vi "S2C_FORNAX_Proc_ProcessReturn.vi"(7 "Text":bool, 8 "Error In":errorcluster, 9 "JSON":string, 10 "Return":string, 11 "Command":string) -> (0 "Error Out":errorcluster, 3 "Data":string)   [LabVIEW 2015]
uses:
  PolyDriver/Typedefs/ParameterRangeState.ctl
  PolyDriver/Typedefs/BoardId.ctl
  PolyDriver/Typedefs/BoardIdDataSet.ctl
  PolyDriver/Typedefs/CalibrationType.ctl
  PolyDriver/Typedefs/ExternalCommPairingStatus.ctl
  PolyDriver/Typedefs/DftMode.ctl
  PolyDriver/Typedefs/SystemSettings.ctl
  PolyDriver/Typedefs/UserSettings.ctl
  PolyDriver/Typedefs/SystemState.ctl
  PolyDriver/Typedefs/EnergyChannelId.ctl
  PolyDriver/Typedefs/EnergyModes.ctl
  PolyDriver/Typedefs/SwitchId.ctl
  PolyDriver/Typedefs/SwitchState.ctl
  PolyDriver/Typedefs/SwitchSource.ctl
  S2C_FORNAX_Proc_Globals.vi
panel:
  in  "SwitchSource":T1 items=["SWITCH_SOURCE_UNKNOWN", "SWITCH_SOURCE_HANDSWITCH", "SWITCH_SOURCE_FOOTSWITCH", "SWITCH_SOURCE_AUTO_BIPOLAR", "SWITCH_SOURCE_CARDIOBLATE", "SWITCH_SOURCE_SCREEN", "NUM_SWITCH_SOURCES"]
  in  "SwitchState":T2 items=["SWITCH_STATE_NULL", "SWITCH_STATE_PRESSED", "SWITCH_STATE_RELEASED", "NUM_SWITCH_STATES"]
  in  "SwitchId":T3 items=["SWITCH_ID_NONE", "SWITCH_ID_CUT", "SWITCH_ID_VMODE", "SWITCH_ID_COAG", "SWITCH_ID_LIGASURE", "SWITCH_ID_BIPOLAR", "SWITCH_ID_STAPLER_CLOSE", "SWITCH_ID_STAPLER_OPEN", "SWITCH_ID_CARDIOBLATE_BIPOLAR", "SWITCH_ID_CARDIOBLATE_BIPOLAR_TOUCHSCREEN", "SWITCH_ID_CARDIOBLATE_MONOPOLAR", "SWITCH_ID_CARDIOBLATE_MONOPOLAR_TOUCHSCREEN", "SWITCH_ID_ULTRASONIC_BTN1", "SWITCH_ID_ULTRASONIC_BTN2", "SWITCH_ID_MAX"]
  in  "EnergyModes":T4 items=["SPRAY_MODE"=0, "CUT_MODE"=1, "BLEND_MODE"=2, "FULGERATE_MODE"=3, "BIPOLAR_MODE"=4, "VESSEL_SEALING_MODE"=5, "VALLEYLAB_MODE"=6, "BIPOLAR_RESECTION_CUT_MODE"=7, "BIPOLAR_RESECTION_COAG_MODE"=8, "AUTOBIPOLAR_MODE"=9, "VIPER_HLA"=10, "SOFT_COAG_MODE"=11, "ECUT_MODE"=12, "SHARED_SPRAY_MODE"=13, "SHARED_FULGERATE_MODE"=14, "CARDIO_MONO_MODE"=15, "CARDIO_BIPOLAR_MODE"=16, "BIPOLAR_LOW_MODE"=17, "BIPOLAR_MACRO_MODE"=18, "BIPOLAR_STANDARD_MODE"=19, "BIPOLAR_MEDIUM_MODE"=20, "VL_ENDOSCOPY_MODE"=21, "NUM_ENERGY_MODES"=22, "MODE_NOT_USED"=-1]
  in  "EnergyChannelId":T5 items=["EC_MONO_1"=0, "EC_BIPOLAR"=1, "EC_MONO_2"=2, "EC_ADVANCED"=3, "EC_ADVANCED_ECUT"=4, "EC_ADVANCED_DCUT"=5, "EC_SHARED_COAG"=6, "EC_INTERNAL_BIP_CAL"=7, "EC_NOT_USED"=-1]
  in  "SystemState":T6 items=["SYSTEM_STATE_INVALID", "SYSTEM_STATE_INIT", "SYSTEM_STATE_POST", "SYSTEM_STATE_CLINICAL", "SYSTEM_STATE_SERVICE", "SYSTEM_STATE_SW_UPDATE", "SYSTEM_STATE_SHUTDOWN", "SYSTEM_STATE_CALIBRATION", "SYSTEM_STATE_CONFIGURATION", "SYSTEM_STATE_CLINICAL_CONFIGURATION"]
  in  "UserSettings":T7 items=["USER_SETTINGS_INVALID", "USER_SETTINGS_LANGUAGE", "USER_SETTINGS_VOLUME", "USER_SETTINGS_ALIAS", "USER_SETTINGS_NETWORK_CONFIG", "USER_SETTINGS_AUTO_NETWORK_ON", "USER_SETTINGS_KEYBOARD_LANGUAGE", "NUM_USER_SETTINGS"]
  in  "SystemSettings":T8 items=["SYSTEM_SETTINGS_INVALID", "SYSTEM_SETTINGS_COUNTRY", "SYSTEM_SETTINGS_REGION", "SYSTEM_SETTINGS_BIPOLAR_RESECTION", "SYSTEM_SETTINGS_INSTRUMENT_ID_MODE", "SYSTEM_SETTINGS_SMOKE_EVAC_MODE", "NUM_SYSTEM_SETTINGS"]
  in  "DftMode":T9 items=["DFT_MODE_NONE", "DFT_MODE_PAIRED", "DFT_MODE_DFA", "DFT_MODE_DFT"]
  in  "ExternalCommPairingStatus":T10 items=["EXTERNAL_COMM_PAIRING_STATUS_NOT_AVAILABLE", "EXTERNAL_COMM_PAIRING_STATUS_AVAILABLE", "EXTERNAL_COMM_PAIRING_STATUS_PAIRED", "NUM_EXTERNAL_COMM_PAIRING_STATUS"]
  in  "CalibrationType":T11 items=["CALIBRATION_TYPE_FIELD"=0, "CALIBRATION_TYPE_FACTORY"=1, "CALIBRATION_TYPE_UNKNOWN"=-1]
  in  "BoardIdDataSet":T12 items=["BOARD_ID_DATASET_BOARD_INFO"=0, "BOARD_ID_DATASET_SCHEMA_INFO"=1, "BOARD_ID_DATASET_CHASSIS_INSTALLATION"=2, "BOARD_ID_DATASET_CONFIGURATION"=3, "BOARD_ID_DATASET_CALIBRATION_CURR"=4, "BOARD_ID_DATASET_RESERVED_1"=5, "BOARD_ID_DATASET_RESERVED_2"=6, "BOARD_ID_DATASET_RESERVED_3"=7, "BOARD_ID_DATASET_CALIBRATION_HIST_TOC"=8, "BOARD_ID_DATASET_CALIBRATION_HIST"=9, "BOARD_ID_DATASET_INIT_MAX"=10, "BOARD_ID_DATASET_MAX"=50]
  in  "BoardId":T13 items=["BOARD_ID_NONE", "BOARD_ID_CONTROLLER", "BOARD_ID_STEERING_RELAY", "BOARD_ID_RF", "BOARD_ID_POWER_SUPPLY", "BOARD_ID_FRONT_PANEL", "BOARD_ID_MAX"]
  in  "ParameterRangeState":T14 items=["PARAMETER_RANGE_STATE_UNKNOWN", "PARAMETER_RANGE_STATE_AT_MIN", "PARAMETER_RANGE_STATE_AT_MAX", "PARAMETER_RANGE_STATE_BETWEEN_MINMAX", "PARAMETER_RANGE_STATE_LESS_THAN_MIN", "PARAMETER_RANGE_STATE_GREATER_THAN_MAX"]
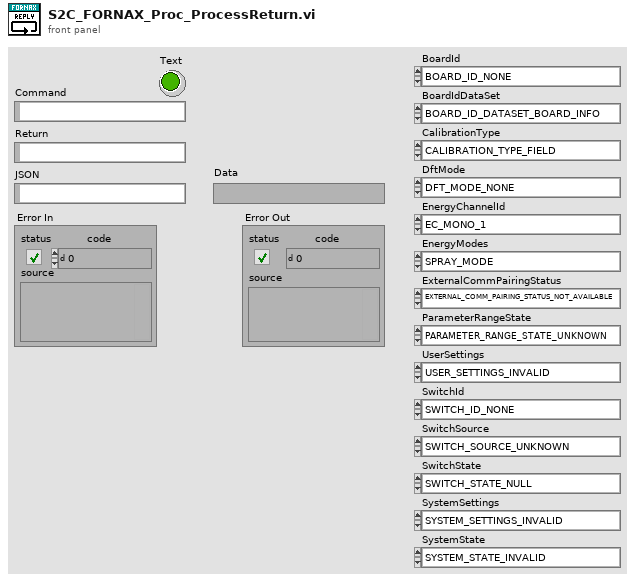
[diagram p1: front panel]
types:
  T1 = typedef "SwitchSource.ctl" = i16
  T2 = typedef "SwitchState.ctl" = i16
  T3 = typedef "SwitchId.ctl" = i16
  T4 = typedef "EnergyModes.ctl" = i16
  T5 = typedef "EnergyChannelId.ctl" = i16
  T6 = typedef "SystemState.ctl" = i16
  T7 = typedef "UserSettings.ctl" = i16
  T8 = typedef "SystemSettings.ctl" = i16
  T9 = typedef "DftMode.ctl" = i16
  T10 = typedef "ExternalCommPairingStatus.ctl" = i16
  T11 = typedef "CalibrationType.ctl" = i16
  T12 = typedef "BoardIdDataSet.ctl" = i16
  T13 = typedef "BoardId.ctl" = i16
  T14 = typedef "ParameterRangeState.ctl" = i16
  T15 = cluster{"Partition":string, "Message":string, "M_BarcodeImageFile":string}
  T16 = cluster{"Partition":string, "Message":string, "M_BoardId":T13, "M_BoardIdDataSet":T12, "M_Value":string, "M_Crc32":i32}
  T17 = cluster{"Partition":string, "Message":string, "M_BoardId":T13, "M_BoardIdDataSet":T12, "M_Value":string}
  T18 = cluster{"Partition":string, "Message":string, "M_EnergyChannelId":T5, "M_CutMode":T4, "M_CutPower":i32, "M_CutPowerRangeState":T14, "M_CoagMode":T4, "M_CoagPower":i32, "M_CoagPowerRangeState":T14, "M_Crc32":i32}
  T19 = cluster{"Partition":string, "Message":string, "M_EnergyChannelId":T5, "M_CutMode":T4, "M_CutPower":i32, "M_CutPowerRangeState":T14, "M_CoagMode":T4, "M_CoagPower":i32, "M_CoagPowerRangeState":T14}
  T20 = cluster{"Partition":string, "Message":string, "M_EnergyChannelId":T5, "M_SourceId":T1, "M_SwitchId":T3, "M_SwitchState":T2, "M_Crc32":i32}
  T21 = cluster{"Partition":string, "Message":string, "M_EnergyChannelId":T5, "M_SourceId":T1, "M_SwitchId":T3, "M_SwitchState":T2}
  T22 = cluster{"Partition":string, "Message":string, "M_CalibrationType":T11, "M_CalibrationTime":string, "M_Options":string, "M_EmA2dCalData.M_MonoLowVoltPrimary.M_Offset":dbl, "M_EmA2dCalData.M_MonoLowVoltPrimary.M_Gain":dbl, "M_EmA2dCalData.M_MonoLowVoltSecondary.M_Offset":dbl, "M_EmA2dCalData.M_MonoLowVoltSecondary.M_Gain":dbl, "M_EmA2dCalData.M_MonoHighVoltPrimary.M_Offset":dbl, "M_EmA2dCalData.M_MonoHighVoltPrimary.M_Gain":dbl, "M_EmA2dCalData.M_MonoHighVoltSecondary.M_Offset":dbl, "M_EmA2dCalData.M_MonoHighVoltSecondary.M_Gain":dbl, "M_EmA2dCalData.M_BipLowVoltPrimary.M_Offset":dbl, "M_EmA2dCalData.M_BipLowVoltPrimary.M_Gain":dbl, "M_EmA2dCalData.M_BipLowVoltSecondary.M_Offset":dbl, "M_EmA2dCalData.M_BipLowVoltSecondary.M_Gain":dbl, "M_EmA2dCalData.M_BipHighVoltPrimary.M_Offset":dbl, "M_EmA2dCalData.M_BipHighVoltPrimary.M_Gain":dbl, "M_EmA2dCalData.M_BipHighVoltSecondary.M_Offset":dbl, "M_EmA2dCalData.M_BipHighVoltSecondary.M_Gain":dbl, "M_EmA2dCalData.M_BipLowCurrentPrimary.M_Offset":dbl, "M_EmA2dCalData.M_BipLowCurrentPrimary.M_Gain":dbl, "M_EmA2dCalData.M_BipLowCurrentSecondary.M_Offset":dbl, "M_EmA2dCalData.M_BipLowCurrentSecondary.M_Gain":dbl, "M_EmA2dCalData.M_BipHighCurrentPrimary.M_Offset":dbl, "M_EmA2dCalData.M_BipHighCurrentPrimary.M_Gain":dbl, "M_EmA2dCalData.M_BipHighCurrentSecondary.M_Offset":dbl, "M_EmA2dCalData.M_BipHighCurrentSecondary.M_Gain":dbl}
  T23 = cluster{"Partition":string, "Message":string, "M_ControllerBoardId":string, "M_ChassisSerialNumber":string, "M_Alias":string, "M_PrimaryIpAddress":string, "M_PairingStatus":T10, "M_PairedEntityIpAddress":string, "M_PairedEntityAlias":string, "M_PairedEntityId":string, "M_Options":string, "M_DftMode":T9, "M_IsViperEnabled":bool}
  T24 = cluster{"Partition":string, "Message":string, "M_DisplayOrder":i32, "M_FeatureSetting":i32, "M_FeatureSettingName":string, "M_FeatureStatus":i32, "M_FeatureStatusText":string, "M_IntValue":i32, "M_IsEnablable":bool, "M_IsEnabled":bool, "M_IsEntitled":bool, "M_IsEntitlable":bool, "M_LastEnabledUpdate":i32, "M_LastEntitledUpdate":i32, "M_LicenseKey":string, "M_LicenseTerms":string, "M_Options":string, "M_StringValue":string}
  T25 = cluster{"Partition":string, "Message":string, "M_SystemSetting":T8, "M_IntValue":i32, "M_StringValue":string}
  T26 = cluster{"Partition":string, "Message":string, "M_UtcTime":string, "M_LocalTime":string, "M_TimeZone":string}
  T27 = cluster{"Partition":string, "Message":string, "M_UserSetting":T7, "M_IntValue":i32, "M_StringValue":string}
  T28 = cluster{"Partition":string, "Message":string, "M_VolumeBars":i32, "M_RangeState":T14, "M_VolumeCloseOverlay":bool}
  T29 = cluster{"Partition":string, "Message":string, "M_ViperMessage":string, "M_SrcId":i32}
  T30 = cluster{"Partition":string, "Message":string, "M_message":string, "M_srcId":i32}
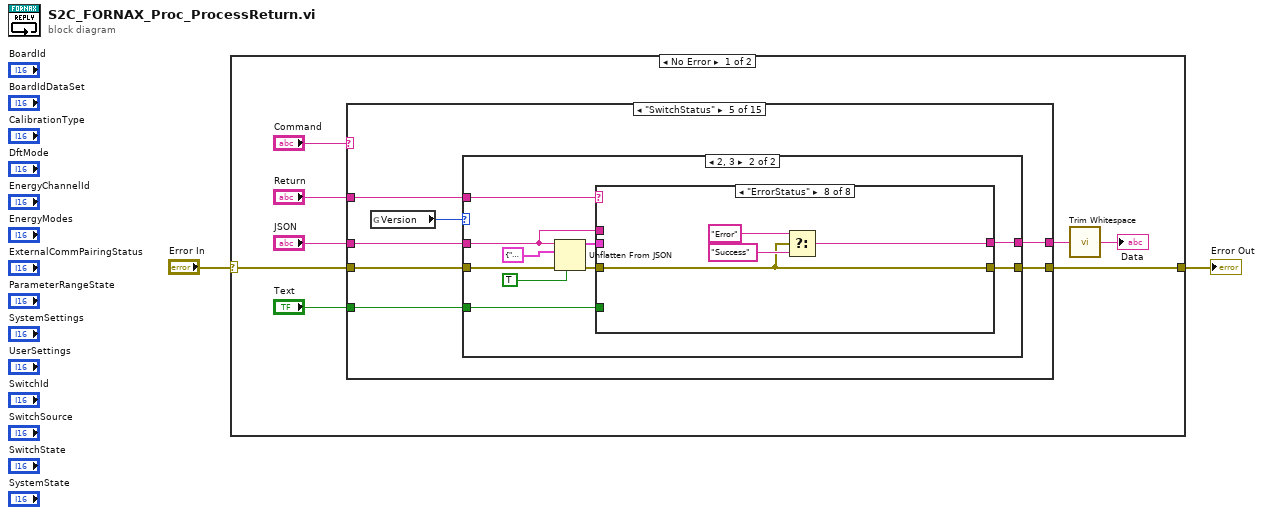
[diagram p0: block diagram]
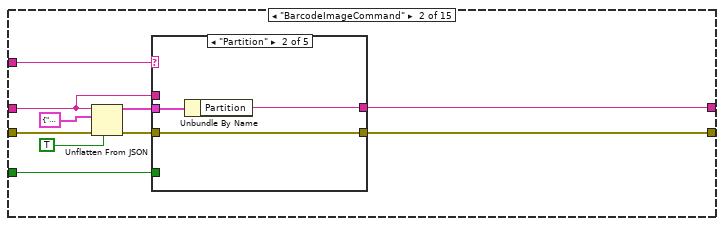
[diagram p3: hidden frame]
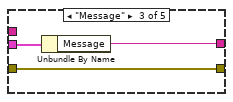
[diagram p5: hidden frame]
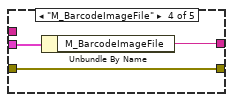
[diagram p6: hidden frame]
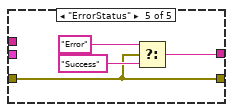
[diagram p7: hidden frame]
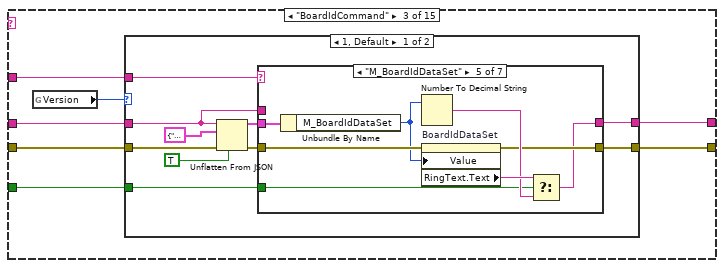
[diagram p8: hidden frame]
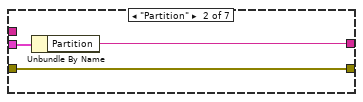
[diagram p10: hidden frame]
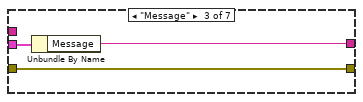
[diagram p11: hidden frame]
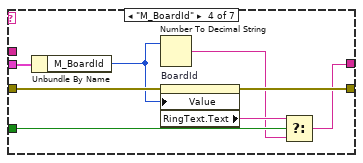
[diagram p12: hidden frame]
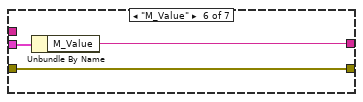
[diagram p13: hidden frame]
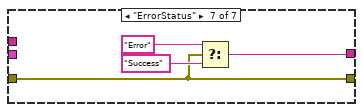
[diagram p14: hidden frame]
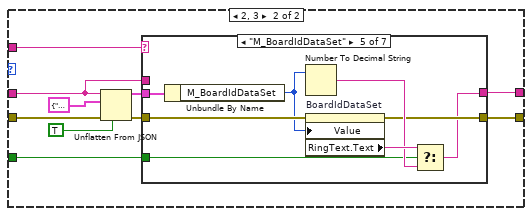
[diagram p15: hidden frame]
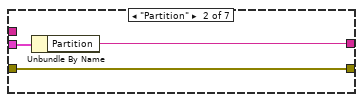
[diagram p17: hidden frame]
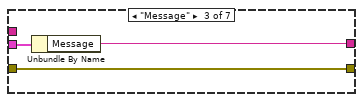
[diagram p18: hidden frame]
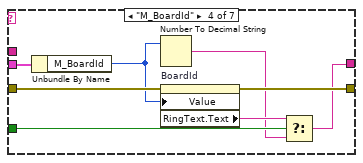
[diagram p19: hidden frame]
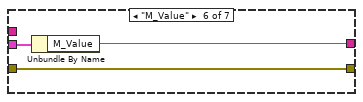
[diagram p20: hidden frame]
diagram:
  n1 = case shown="No Error" "Error In" {
    selector: "Error In" -> [w10 w919]
    tunnel: [w5 w919] -> w1
    frame No Error {
      n2 = case shown="\"SwitchStatus\"" "Command" {
        tunnel: w10 -> [w12 w22 w44 w133 w284 w406 w538 w606 w685 w697 w718 w755 w786 w823 w860]
        tunnel: "Return" -> [_ w19 w43 w132 w283 w403 w535 w603 w690 w702 w715 w752 w783 w820 w859]
        tunnel: "JSON" -> [w11 w17 w42 w131 w282 w401 w533 w601 w689 w701 w713 w750 w781 w818 w858]
        tunnel: [w11 w16 w41 w130 w281 w400 w532 w600 w688 w700 w712 w749 w780 w817 w857] -> w6
        tunnel: [w12 w15 w40 w129 w280 w399 w531 w599 w687 w699 w711 w748 w779 w816 w856] -> w5
        tunnel: "Text" -> [_ w14 w39 w128 w279 w398 w530 w598 w686 w698 w710 w747 w778 w815 w855]
        frame "Unknown", Default {
        }
        frame "BarcodeImageCommand" {
          n3 = Unflatten From JSON(JSON string=w17, type and defaults=T15 {"Partition"="", "Message"="", "M_BarcodeImageFile"=""}, default null elements? (F)=TRUE, error in (no error)=w22) -> (value=w18:T15, error out=w20:errorcluster)  [unwired: 3 in]
          n4 = case shown="\"Partition\"" w19 {
            tunnel: w20 -> [w23 w25 w28 w31 w34]
            tunnel: w18 -> [_ w27 w30 w33 _]
            tunnel: w17 -> [w24 _ _ _ _]
            tunnel: [w24 w26 w29 w32 w35] -> w16
            tunnel: [w23 w25 w28 w31 w34] -> w15
            tunnel: w14 -> [_ _ _ _ _]
            frame "All", Default {
            }
            frame "Partition" {
              n5 = Unbundle By Name(w27) -> ("Partition"=w26:string)
            }
            frame "Message" {
              n6 = Unbundle By Name(w30) -> ("Message"=w29:string)
            }
            frame "M_BarcodeImageFile" {
              n7 = Unbundle By Name(w33) -> ("M_BarcodeImageFile"=w32:string)
            }
            frame "ErrorStatus" {
              n8 = Select(t="Error", s=w34, f="Success") -> (s? t:f=w35:string)
            }
          }
        }
        frame "BoardIdCommand" {
          n9 = global read "S2C_FORNAX_Proc_Globals.vi" "Version"() -> (w38:i32)
          n10 = case shown="1, Default" w38 {
            tunnel: w44 -> [w54 w95]
            tunnel: w43 -> [w51 w92]
            tunnel: w42 -> [w49 w90]
            tunnel: [w48 w89] -> w41
            tunnel: [w47 w88] -> w40
            tunnel: w39 -> [w46 w87]
            frame 1, Default {
              n11 = Unflatten From JSON(JSON string=w49, type and defaults=T16 {"Partition"="", "Message"="", "M_BoardId"=0, "M_BoardIdDataSet"=50, "M_Value"="", "M_Crc32"=0}, default null elements? (F)=TRUE, error in (no error)=w54) -> (value=w50:T16, error out=w52:errorcluster)  [unwired: 3 in]
              n12 = case shown="\"M_BoardIdDataSet\"" w51 {
                tunnel: w52 -> [w55 w57 w60 w69 w75 w79 w82]
                tunnel: w50 -> [_ w59 w62 w70 w78 w81 _]
                tunnel: w49 -> [w56 _ _ _ _ _ _]
                tunnel: [w56 w58 w61 w63 w73 w80 w83] -> w48
                tunnel: [w55 w57 w60 w68 w74 w79 w82] -> w47
                tunnel: w46 -> [_ _ _ w65 w71 _ _]
                frame "All", Default {
                }
                frame "Partition" {
                  n13 = Unbundle By Name(w59) -> ("Partition"=w58:string)
                }
                frame "Message" {
                  n14 = Unbundle By Name(w62) -> ("Message"=w61:string)
                }
                frame "M_BoardId" {
                  n15 = Unbundle By Name(w70) -> ("M_BoardId"=w66:T13)
                  n16 = Number To Decimal String(number=w66) -> (decimal integer string=w64:string)  [unwired: 1 in]
                  n17 = property on="BoardId" class="Ring (strict)"(error in=w69, "Value"=w66) -> (error out=w68:errorcluster, "RingText.Text"=w67:string)  [unwired: 1 in, 1 out]
                  n18 = Select(t=w67, s=w65, f=w64) -> (s? t:f=w63:string)
                }
                frame "M_BoardIdDataSet" {
                  n19 = Unbundle By Name(w78) -> ("M_BoardIdDataSet"=w72:T12)
                  n20 = Number To Decimal String(number=w72) -> (decimal integer string=w76:string)  [unwired: 1 in]
                  n21 = property on="BoardIdDataSet" class="Ring (strict)"(error in=w75, "Value"=w72) -> (error out=w74:errorcluster, "RingText.Text"=w77:string)  [unwired: 1 in, 1 out]
                  n22 = Select(t=w77, s=w71, f=w76) -> (s? t:f=w73:string)
                }
                frame "M_Value" {
                  n23 = Unbundle By Name(w81) -> ("M_Value"=w80:string)
                }
                frame "ErrorStatus" {
                  n24 = Select(t="Error", s=w82, f="Success") -> (s? t:f=w83:string)
                }
              }
            }
            frame 2, 3 {
              n25 = Unflatten From JSON(JSON string=w90, type and defaults=T17 {"Partition"="", "Message"="", "M_BoardId"=0, "M_BoardIdDataSet"=50, "M_Value"=""}, default null elements? (F)=TRUE, error in (no error)=w95) -> (value=w91:T17, error out=w93:errorcluster)  [unwired: 3 in]
              n26 = case shown="\"M_BoardIdDataSet\"" w92 {
                tunnel: w93 -> [w96 w98 w101 w110 w116 w120 w123]
                tunnel: w91 -> [_ w100 w103 w111 w119 w122 _]
                tunnel: w90 -> [w97 _ _ _ _ _ _]
                tunnel: [w97 w99 w102 w104 w114 w121 w124] -> w89
                tunnel: [w96 w98 w101 w109 w115 w120 w123] -> w88
                tunnel: w87 -> [_ _ _ w106 w112 _ _]
                frame "All", Default {
                }
                frame "Partition" {
                  n27 = Unbundle By Name(w100) -> ("Partition"=w99:string)
                }
                frame "Message" {
                  n28 = Unbundle By Name(w103) -> ("Message"=w102:string)
                }
                frame "M_BoardId" {
                  n29 = Unbundle By Name(w111) -> ("M_BoardId"=w107:T13)
                  n30 = Number To Decimal String(number=w107) -> (decimal integer string=w105:string)  [unwired: 1 in]
                  n31 = property on="BoardId" class="Ring (strict)"(error in=w110, "Value"=w107) -> (error out=w109:errorcluster, "RingText.Text"=w108:string)  [unwired: 1 in, 1 out]
                  n32 = Select(t=w108, s=w106, f=w105) -> (s? t:f=w104:string)
                }
                frame "M_BoardIdDataSet" {
                  n33 = Unbundle By Name(w119) -> ("M_BoardIdDataSet"=w113:T12)
                  n34 = Number To Decimal String(number=w113) -> (decimal integer string=w117:string)  [unwired: 1 in]
                  n35 = property on="BoardIdDataSet" class="Ring (strict)"(error in=w116, "Value"=w113) -> (error out=w115:errorcluster, "RingText.Text"=w118:string)  [unwired: 1 in, 1 out]
                  n36 = Select(t=w118, s=w112, f=w117) -> (s? t:f=w114:string)
                }
                frame "M_Value" {
                  n37 = Unbundle By Name(w122) -> ("M_Value"=w121:string)
                }
                frame "ErrorStatus" {
                  n38 = Select(t="Error", s=w123, f="Success") -> (s? t:f=w124:string)
                }
              }
            }
          }
        }
        frame "MonopolarCommand" {
          n39 = global read "S2C_FORNAX_Proc_Globals.vi" "Version"() -> (w127:i32)
          n40 = case shown="2, 3" w127 {
            tunnel: w133 -> [w143 w217]
            tunnel: w132 -> [w140 w214]
            tunnel: w131 -> [w138 w212]
            tunnel: [w137 w211] -> w130
            tunnel: [w136 w210] -> w129
            tunnel: w128 -> [w135 w209]
            frame 1, Default {
              n41 = Unflatten From JSON(JSON string=w138, type and defaults=T18 {"Partition"="", "Message"="", "M_EnergyChannelId"=0, "M_CutMode"=0, "M_CutPower"=0, "M_CutPowerRangeState"=0, "M_CoagMode"=0, "M_CoagPower"=0, "M_CoagPowerRangeState"=0, "M_Crc32"=0}, default null elements? (F)=TRUE, error in (no error)=w143) -> (value=w139:T18, error out=w141:errorcluster)  [unwired: 3 in]
              n42 = case shown="\"ErrorStatus\"" w140 {
                tunnel: w141 -> [w144 w146 w149 w158 w164 w170 w176 w184 w190 w196 w202 w204]
                tunnel: w139 -> [_ w148 w151 w159 w167 w171 w179 w187 w191 w199 w203 _]
                tunnel: w138 -> [w145 _ _ _ _ _ _ _ _ _ _ _]
                tunnel: [w145 w147 w150 w152 w162 w168 w174 w182 w188 w194 w200 w205] -> w137
                tunnel: [w144 w146 w149 w157 w163 w170 w175 w183 w190 w195 w202 w204] -> w136
                tunnel: w135 -> [_ _ _ w154 w160 _ w172 w180 _ w192 _ _]
                frame "All", Default {
                }
                frame "Partition" {
                  n43 = Unbundle By Name(w148) -> ("Partition"=w147:string)
                }
                frame "Message" {
                  n44 = Unbundle By Name(w151) -> ("Message"=w150:string)
                }
                frame "M_EnergyChannelId" {
                  n45 = Unbundle By Name(w159) -> ("M_EnergyChannelId"=w155:T5)
                  n46 = Number To Decimal String(number=w155) -> (decimal integer string=w153:string)  [unwired: 1 in]
                  n47 = property on="EnergyChannelId" class="Ring (strict)"(error in=w158, "Value"=w155) -> (error out=w157:errorcluster, "RingText.Text"=w156:string)  [unwired: 1 in, 1 out]
                  n48 = Select(t=w156, s=w154, f=w153) -> (s? t:f=w152:string)
                }
                frame "M_CutMode" {
                  n49 = Unbundle By Name(w167) -> ("M_CutMode"=w161:T4)
                  n50 = Number To Decimal String(number=w161) -> (decimal integer string=w165:string)  [unwired: 1 in]
                  n51 = property on="EnergyModes" class="Ring (strict)"(error in=w164, "Value"=w161) -> (error out=w163:errorcluster, "RingText.Text"=w166:string)  [unwired: 1 in, 1 out]
                  n52 = Select(t=w166, s=w160, f=w165) -> (s? t:f=w162:string)
                }
                frame "M_CutPower" {
                  n53 = Unbundle By Name(w171) -> ("M_CutPower"=w169:i32)
                  n54 = Number To Decimal String(number=w169) -> (decimal integer string=w168:string)  [unwired: 1 in]
                }
                frame "M_CutPowerRangeState" {
                  n55 = Unbundle By Name(w179) -> ("M_CutPowerRangeState"=w173:T14)
                  n56 = Number To Decimal String(number=w173) -> (decimal integer string=w177:string)  [unwired: 1 in]
                  n57 = property on="ParameterRangeState" class="Ring (strict)"(error in=w176, "Value"=w173) -> (error out=w175:errorcluster, "RingText.Text"=w178:string)  [unwired: 1 in, 1 out]
                  n58 = Select(t=w178, s=w172, f=w177) -> (s? t:f=w174:string)
                }
                frame "M_CoagMode" {
                  n59 = Unbundle By Name(w187) -> ("M_CoagMode"=w181:T4)
                  n60 = Number To Decimal String(number=w181) -> (decimal integer string=w185:string)  [unwired: 1 in]
                  n61 = property on="EnergyModes" class="Ring (strict)"(error in=w184, "Value"=w181) -> (error out=w183:errorcluster, "RingText.Text"=w186:string)  [unwired: 1 in, 1 out]
                  n62 = Select(t=w186, s=w180, f=w185) -> (s? t:f=w182:string)
                }
                frame "M_CoagPower" {
                  n63 = Unbundle By Name(w191) -> ("M_CoagPower"=w189:i32)
                  n64 = Number To Decimal String(number=w189) -> (decimal integer string=w188:string)  [unwired: 1 in]
                }
                frame "M_CoagPowerRangeState" {
                  n65 = Unbundle By Name(w199) -> ("M_CoagPowerRangeState"=w193:T14)
                  n66 = Number To Decimal String(number=w193) -> (decimal integer string=w197:string)  [unwired: 1 in]
                  n67 = property on="ParameterRangeState" class="Ring (strict)"(error in=w196, "Value"=w193) -> (error out=w195:errorcluster, "RingText.Text"=w198:string)  [unwired: 1 in, 1 out]
                  n68 = Select(t=w198, s=w192, f=w197) -> (s? t:f=w194:string)
                }
                frame "M_Crc32" {
                  n69 = Unbundle By Name(w203) -> ("M_Crc32"=w201:i32)
                  n70 = Number To Decimal String(number=w201) -> (decimal integer string=w200:string)  [unwired: 1 in]
                }
                frame "ErrorStatus" {
                  n71 = Select(t="Error", s=w204, f="Success") -> (s? t:f=w205:string)
                }
              }
            }
            frame 2, 3 {
              n72 = Unflatten From JSON(JSON string=w212, type and defaults=T19 {"Partition"="", "Message"="", "M_EnergyChannelId"=0, "M_CutMode"=0, "M_CutPower"=0, "M_CutPowerRangeState"=0, "M_CoagMode"=0, "M_CoagPower"=0, "M_CoagPowerRangeState"=0}, default null elements? (F)=TRUE, error in (no error)=w217) -> (value=w213:T19, error out=w215:errorcluster)  [unwired: 3 in]
              n73 = case shown="\"ErrorStatus\"" w214 {
                tunnel: w215 -> [w218 w220 w223 w232 w238 w244 w250 w258 w264 w270 w274]
                tunnel: w213 -> [_ w222 w225 w233 w241 w245 w253 w261 w265 w273 _]
                tunnel: w212 -> [w219 _ _ _ _ _ _ _ _ _ _]
                tunnel: [w219 w221 w224 w226 w236 w242 w248 w256 w262 w268 w275] -> w211
                tunnel: [w218 w220 w223 w231 w237 w244 w249 w257 w264 w269 w274] -> w210
                tunnel: w209 -> [_ _ _ w228 w234 _ w246 w254 _ w266 _]
                frame "All", Default {
                }
                frame "Partition" {
                  n74 = Unbundle By Name(w222) -> ("Partition"=w221:string)
                }
                frame "Message" {
                  n75 = Unbundle By Name(w225) -> ("Message"=w224:string)
                }
                frame "M_EnergyChannelId" {
                  n76 = Unbundle By Name(w233) -> ("M_EnergyChannelId"=w229:T5)
                  n77 = Number To Decimal String(number=w229) -> (decimal integer string=w227:string)  [unwired: 1 in]
                  n78 = property on="EnergyChannelId" class="Ring (strict)"(error in=w232, "Value"=w229) -> (error out=w231:errorcluster, "RingText.Text"=w230:string)  [unwired: 1 in, 1 out]
                  n79 = Select(t=w230, s=w228, f=w227) -> (s? t:f=w226:string)
                }
                frame "M_CutMode" {
                  n80 = Unbundle By Name(w241) -> ("M_CutMode"=w235:T4)
                  n81 = Number To Decimal String(number=w235) -> (decimal integer string=w239:string)  [unwired: 1 in]
                  n82 = property on="EnergyModes" class="Ring (strict)"(error in=w238, "Value"=w235) -> (error out=w237:errorcluster, "RingText.Text"=w240:string)  [unwired: 1 in, 1 out]
                  n83 = Select(t=w240, s=w234, f=w239) -> (s? t:f=w236:string)
                }
                frame "M_CutPower" {
                  n84 = Unbundle By Name(w245) -> ("M_CutPower"=w243:i32)
                  n85 = Number To Decimal String(number=w243) -> (decimal integer string=w242:string)  [unwired: 1 in]
                }
                frame "M_CutPowerRangeState" {
                  n86 = Unbundle By Name(w253) -> ("M_CutPowerRangeState"=w247:T14)
                  n87 = Number To Decimal String(number=w247) -> (decimal integer string=w251:string)  [unwired: 1 in]
                  n88 = property on="ParameterRangeState" class="Ring (strict)"(error in=w250, "Value"=w247) -> (error out=w249:errorcluster, "RingText.Text"=w252:string)  [unwired: 1 in, 1 out]
                  n89 = Select(t=w252, s=w246, f=w251) -> (s? t:f=w248:string)
                }
                frame "M_CoagMode" {
                  n90 = Unbundle By Name(w261) -> ("M_CoagMode"=w255:T4)
                  n91 = Number To Decimal String(number=w255) -> (decimal integer string=w259:string)  [unwired: 1 in]
                  n92 = property on="EnergyModes" class="Ring (strict)"(error in=w258, "Value"=w255) -> (error out=w257:errorcluster, "RingText.Text"=w260:string)  [unwired: 1 in, 1 out]
                  n93 = Select(t=w260, s=w254, f=w259) -> (s? t:f=w256:string)
                }
                frame "M_CoagPower" {
                  n94 = Unbundle By Name(w265) -> ("M_CoagPower"=w263:i32)
                  n95 = Number To Decimal String(number=w263) -> (decimal integer string=w262:string)  [unwired: 1 in]
                }
                frame "M_CoagPowerRangeState" {
                  n96 = Unbundle By Name(w273) -> ("M_CoagPowerRangeState"=w267:T14)
                  n97 = Number To Decimal String(number=w267) -> (decimal integer string=w271:string)  [unwired: 1 in]
                  n98 = property on="ParameterRangeState" class="Ring (strict)"(error in=w270, "Value"=w267) -> (error out=w269:errorcluster, "RingText.Text"=w272:string)  [unwired: 1 in, 1 out]
                  n99 = Select(t=w272, s=w266, f=w271) -> (s? t:f=w268:string)
                }
                frame "ErrorStatus" {
                  n100 = Select(t="Error", s=w274, f="Success") -> (s? t:f=w275:string)
                }
              }
            }
          }
        }
        frame "SwitchStatus" {
          n101 = global read "S2C_FORNAX_Proc_Globals.vi" "Version"() -> (w278:i32)
          n102 = case shown="2, 3" w278 {
            tunnel: w284 -> [w294 w352]
            tunnel: w283 -> [w291 w349]
            tunnel: w282 -> [w289 w347]
            tunnel: [w288 w346] -> w281
            tunnel: [w287 w345] -> w280
            tunnel: w279 -> [w286 w344]
            frame 1, Default {
              n103 = Unflatten From JSON(JSON string=w289, type and defaults=T20 {"Partition"="", "Message"="", "M_EnergyChannelId"=0, "M_SourceId"=0, "M_SwitchId"=0, "M_SwitchState"=0, "M_Crc32"=0}, default null elements? (F)=TRUE, error in (no error)=w294) -> (value=w290:T20, error out=w292:errorcluster)  [unwired: 3 in]
              n104 = case shown="\"M_Crc32\"" w291 {
                tunnel: w292 -> [w295 w297 w300 w309 w315 w323 w331 w337 w339]
                tunnel: w290 -> [_ w299 w302 w310 w318 w326 w334 w338 _]
                tunnel: w289 -> [w296 _ _ _ _ _ _ _ _]
                tunnel: [w296 w298 w301 w303 w313 w321 w329 w335 w340] -> w288
                tunnel: [w295 w297 w300 w308 w314 w322 w330 w337 w339] -> w287
                tunnel: w286 -> [_ _ _ w305 w311 w319 w327 _ _]
                frame "All", Default {
                }
                frame "Partition" {
                  n105 = Unbundle By Name(w299) -> ("Partition"=w298:string)
                }
                frame "Message" {
                  n106 = Unbundle By Name(w302) -> ("Message"=w301:string)
                }
                frame "M_EnergyChannelId" {
                  n107 = Unbundle By Name(w310) -> ("M_EnergyChannelId"=w306:T5)
                  n108 = Number To Decimal String(number=w306) -> (decimal integer string=w304:string)  [unwired: 1 in]
                  n109 = property on="EnergyChannelId" class="Ring (strict)"(error in=w309, "Value"=w306) -> (error out=w308:errorcluster, "RingText.Text"=w307:string)  [unwired: 1 in, 1 out]
                  n110 = Select(t=w307, s=w305, f=w304) -> (s? t:f=w303:string)
                }
                frame "M_SourceId" {
                  n111 = Unbundle By Name(w318) -> ("M_SourceId"=w312:T1)
                  n112 = Number To Decimal String(number=w312) -> (decimal integer string=w316:string)  [unwired: 1 in]
                  n113 = property on="SwitchSource" class="Ring (strict)"(error in=w315, "Value"=w312) -> (error out=w314:errorcluster, "RingText.Text"=w317:string)  [unwired: 1 in, 1 out]
                  n114 = Select(t=w317, s=w311, f=w316) -> (s? t:f=w313:string)
                }
                frame "M_SwitchId" {
                  n115 = Unbundle By Name(w326) -> ("M_SwitchId"=w320:T3)
                  n116 = Number To Decimal String(number=w320) -> (decimal integer string=w324:string)  [unwired: 1 in]
                  n117 = property on="SwitchId" class="Ring (strict)"(error in=w323, "Value"=w320) -> (error out=w322:errorcluster, "RingText.Text"=w325:string)  [unwired: 1 in, 1 out]
                  n118 = Select(t=w325, s=w319, f=w324) -> (s? t:f=w321:string)
                }
                frame "M_SwitchState" {
                  n119 = Unbundle By Name(w334) -> ("M_SwitchState"=w328:T2)
                  n120 = Number To Decimal String(number=w328) -> (decimal integer string=w332:string)  [unwired: 1 in]
                  n121 = property on="SwitchState" class="Ring (strict)"(error in=w331, "Value"=w328) -> (error out=w330:errorcluster, "RingText.Text"=w333:string)  [unwired: 1 in, 1 out]
                  n122 = Select(t=w333, s=w327, f=w332) -> (s? t:f=w329:string)
                }
                frame "M_Crc32" {
                  n123 = Unbundle By Name(w338) -> ("M_Crc32"=w336:i32)
                  n124 = Number To Decimal String(number=w336) -> (decimal integer string=w335:string)  [unwired: 1 in]
                }
                frame "ErrorStatus" {
                  n125 = Select(t="Error", s=w339, f="Success") -> (s? t:f=w340:string)
                }
              }
            }
            frame 2, 3 {
              n126 = Unflatten From JSON(JSON string=w347, type and defaults=T21 {"Partition"="", "Message"="", "M_EnergyChannelId"=0, "M_SourceId"=0, "M_SwitchId"=0, "M_SwitchState"=0}, default null elements? (F)=TRUE, error in (no error)=w352) -> (value=w348:T21, error out=w350:errorcluster)  [unwired: 3 in]
              n127 = case shown="\"ErrorStatus\"" w349 {
                tunnel: w350 -> [w353 w355 w358 w367 w373 w381 w389 w393]
                tunnel: w348 -> [_ w357 w360 w368 w376 w384 w392 _]
                tunnel: w347 -> [w354 _ _ _ _ _ _ _]
                tunnel: [w354 w356 w359 w361 w371 w379 w387 w394] -> w346
                tunnel: [w353 w355 w358 w366 w372 w380 w388 w393] -> w345
                tunnel: w344 -> [_ _ _ w363 w369 w377 w385 _]
                frame "All", Default {
                }
                frame "Partition" {
                  n128 = Unbundle By Name(w357) -> ("Partition"=w356:string)
                }
                frame "Message" {
                  n129 = Unbundle By Name(w360) -> ("Message"=w359:string)
                }
                frame "M_EnergyChannelId" {
                  n130 = Unbundle By Name(w368) -> ("M_EnergyChannelId"=w364:T5)
                  n131 = Number To Decimal String(number=w364) -> (decimal integer string=w362:string)  [unwired: 1 in]
                  n132 = property on="EnergyChannelId" class="Ring (strict)"(error in=w367, "Value"=w364) -> (error out=w366:errorcluster, "RingText.Text"=w365:string)  [unwired: 1 in, 1 out]
                  n133 = Select(t=w365, s=w363, f=w362) -> (s? t:f=w361:string)
                }
                frame "M_SourceId" {
                  n134 = Unbundle By Name(w376) -> ("M_SourceId"=w370:T1)
                  n135 = Number To Decimal String(number=w370) -> (decimal integer string=w374:string)  [unwired: 1 in]
                  n136 = property on="SwitchSource" class="Ring (strict)"(error in=w373, "Value"=w370) -> (error out=w372:errorcluster, "RingText.Text"=w375:string)  [unwired: 1 in, 1 out]
                  n137 = Select(t=w375, s=w369, f=w374) -> (s? t:f=w371:string)
                }
                frame "M_SwitchId" {
                  n138 = Unbundle By Name(w384) -> ("M_SwitchId"=w378:T3)
                  n139 = Number To Decimal String(number=w378) -> (decimal integer string=w382:string)  [unwired: 1 in]
                  n140 = property on="SwitchId" class="Ring (strict)"(error in=w381, "Value"=w378) -> (error out=w380:errorcluster, "RingText.Text"=w383:string)  [unwired: 1 in, 1 out]
                  n141 = Select(t=w383, s=w377, f=w382) -> (s? t:f=w379:string)
                }
                frame "M_SwitchState" {
                  n142 = Unbundle By Name(w392) -> ("M_SwitchState"=w386:T2)
                  n143 = Number To Decimal String(number=w386) -> (decimal integer string=w390:string)  [unwired: 1 in]
                  n144 = property on="SwitchState" class="Ring (strict)"(error in=w389, "Value"=w386) -> (error out=w388:errorcluster, "RingText.Text"=w391:string)  [unwired: 1 in, 1 out]
                  n145 = Select(t=w391, s=w385, f=w390) -> (s? t:f=w387:string)
                }
                frame "ErrorStatus" {
                  n146 = Select(t="Error", s=w393, f="Success") -> (s? t:f=w394:string)
                }
              }
            }
          }
        }
        frame "EmA2dCalDataCommand" {
          n147 = Unflatten From JSON(JSON string=w401, type and defaults=T22 {"Partition"="", "Message"="", "M_CalibrationType"=0, "M_CalibrationTime"="", "M_Options"="", "M_EmA2dCalData.M_MonoLowVoltPrimary.M_Offset"=0.0, "M_EmA2dCalData.M_MonoLowVoltPrimary.M_Gain"=0.0, "M_EmA2dCalData.M_MonoLowVoltSecondary.M_Offset"=0.0, "M_EmA2dCalData.M_MonoLowVoltSecondary.M_Gain"=0.0, "M_EmA2dCalData.M_MonoHighVoltPrimary.M_Offset"=0.0, "M_EmA2dCalData.M_MonoHighVoltPrimary.M_Gain"=0.0, "M_EmA2dCalData.M_MonoHighVoltSecondary.M_Offset"=0.0, "M_EmA2dCalData.M_MonoHighVoltSecondary.M_Gain"=0.0, "M_EmA2dCalData.M_BipLowVoltPrimary.M_Offset"=0.0, "M_EmA2dCalData.M_BipLowVoltPrimary.M_Gain"=0.0, "M_EmA2dCalData.M_BipLowVoltSecondary.M_Offset"=0.0, "M_EmA2dCalData.M_BipLowVoltSecondary.M_Gain"=0.0, "M_EmA2dCalData.M_BipHighVoltPrimary.M_Offset"=0.0, "M_EmA2dCalData.M_BipHighVoltPrimary.M_Gain"=0.0, "M_EmA2dCalData.M_BipHighVoltSecondary.M_Offset"=0.0, "M_EmA2dCalData.M_BipHighVoltSecondary.M_Gain"=0.0, "M_EmA2dCalData.M_BipLowCurrentPrimary.M_Offset"=0.0, "M_EmA2dCalData.M_BipLowCurrentPrimary.M_Gain"=0.0, "M_EmA2dCalData.M_BipLowCurrentSecondary.M_Offset"=0.0, "M_EmA2dCalData.M_BipLowCurrentSecondary.M_Gain"=0.0, "M_EmA2dCalData.M_BipHighCurrentPrimary.M_Offset"=0.0, "M_EmA2dCalData.M_BipHighCurrentPrimary.M_Gain"=0.0, "M_EmA2dCalData.M_BipHighCurrentSecondary.M_Offset"=0.0, "M_EmA2dCalData.M_BipHighCurrentSecondary.M_Gain"=0.0}, default null elements? (F)=TRUE, error in (no error)=w406) -> (value=w402:T22, error out=w404:errorcluster)  [unwired: 3 in]
          n148 = case shown="\"ErrorStatus\"" w403 {
            tunnel: w404 -> [w407 w409 w412 w421 w423 w426 w431 w435 w439 w443 w447 w451 w455 w459 w463 w467 w471 w475 w479 w483 w487 w491 w495 w499 w503 w507 w511 w515 w519 w523 w525]
            tunnel: w402 -> [_ w411 w414 w422 w425 w428 w432 w436 w440 w444 w448 w452 w456 w460 w464 w468 w472 w476 w480 w484 w488 w492 w496 w500 w504 w508 w512 w516 w520 w524 _]
            tunnel: w401 -> [w408 _ _ _ _ _ _ _ _ _ _ _ _ _ _ _ _ _ _ _ _ _ _ _ _ _ _ _ _ _ _]
            tunnel: [w408 w410 w413 w415 w424 w427 w429 w433 w437 w441 w445 w449 w453 w457 w461 w465 w469 w473 w477 w481 w485 w489 w493 w497 w501 w505 w509 w513 w517 w521 w526] -> w400
            tunnel: [w407 w409 w412 w420 w423 w426 w431 w435 w439 w443 w447 w451 w455 w459 w463 w467 w471 w475 w479 w483 w487 w491 w495 w499 w503 w507 w511 w515 w519 w523 w525] -> w399
            tunnel: w398 -> [_ _ _ w417 _ _ _ _ _ _ _ _ _ _ _ _ _ _ _ _ _ _ _ _ _ _ _ _ _ _ _]
            frame "All", Default {
            }
            frame "Partition" {
              n149 = Unbundle By Name(w411) -> ("Partition"=w410:string)
            }
            frame "Message" {
              n150 = Unbundle By Name(w414) -> ("Message"=w413:string)
            }
            frame "M_CalibrationType" {
              n151 = Unbundle By Name(w422) -> ("M_CalibrationType"=w418:T11)
              n152 = Number To Decimal String(number=w418) -> (decimal integer string=w416:string)  [unwired: 1 in]
              n153 = property on="BoardId" class="Ring (strict)"(error in=w421, "Value"=w418) -> (error out=w420:errorcluster, "RingText.Text"=w419:string)  [unwired: 1 in, 1 out]
              n154 = Select(t=w419, s=w417, f=w416) -> (s? t:f=w415:string)
            }
            frame "M_CalibrationTime" {
              n155 = Unbundle By Name(w425) -> ("M_CalibrationTime"=w424:string)
            }
            frame "M_Options" {
              n156 = Unbundle By Name(w428) -> ("M_Options"=w427:string)
            }
            frame "M_EmA2dCalData.M_MonoLowVoltPrimary.M_Offset" {
              n157 = Unbundle By Name(w432) -> ("M_EmA2dCalData.M_MonoLowVoltPrimary.M_Offset"=w430:dbl)
              n158 = Number To Fractional String(number=w430) -> (F-format string=w429:string)  [unwired: 3 in]
            }
            frame "M_EmA2dCalData.M_MonoLowVoltPrimary.M_Gain" {
              n159 = Unbundle By Name(w436) -> ("M_EmA2dCalData.M_MonoLowVoltPrimary.M_Gain"=w434:dbl)
              n160 = Number To Fractional String(number=w434) -> (F-format string=w433:string)  [unwired: 3 in]
            }
            frame "M_EmA2dCalData.M_MonoLowVoltSecondary.M_Offset" {
              n161 = Unbundle By Name(w440) -> ("M_EmA2dCalData.M_MonoLowVoltSecondary.M_Offset"=w438:dbl)
              n162 = Number To Fractional String(number=w438) -> (F-format string=w437:string)  [unwired: 3 in]
            }
            frame "M_EmA2dCalData.M_MonoLowVoltSecondary.M_Gain" {
              n163 = Unbundle By Name(w444) -> ("M_EmA2dCalData.M_MonoLowVoltSecondary.M_Gain"=w442:dbl)
              n164 = Number To Fractional String(number=w442) -> (F-format string=w441:string)  [unwired: 3 in]
            }
            frame "M_EmA2dCalData.M_MonoHighVoltPrimary.M_Offset" {
              n165 = Unbundle By Name(w448) -> ("M_EmA2dCalData.M_MonoHighVoltPrimary.M_Offset"=w446:dbl)
              n166 = Number To Fractional String(number=w446) -> (F-format string=w445:string)  [unwired: 3 in]
            }
            frame "M_EmA2dCalData.M_MonoHighVoltPrimary.M_Gain" {
              n167 = Unbundle By Name(w452) -> ("M_EmA2dCalData.M_MonoHighVoltPrimary.M_Gain"=w450:dbl)
              n168 = Number To Fractional String(number=w450) -> (F-format string=w449:string)  [unwired: 3 in]
            }
            frame "M_EmA2dCalData.M_MonoHighVoltSecondary.M_Offset" {
              n169 = Unbundle By Name(w456) -> ("M_EmA2dCalData.M_MonoHighVoltSecondary.M_Offset"=w454:dbl)
              n170 = Number To Fractional String(number=w454) -> (F-format string=w453:string)  [unwired: 3 in]
            }
            frame "M_EmA2dCalData.M_MonoHighVoltSecondary.M_Gain" {
              n171 = Unbundle By Name(w460) -> ("M_EmA2dCalData.M_MonoHighVoltSecondary.M_Gain"=w458:dbl)
              n172 = Number To Fractional String(number=w458) -> (F-format string=w457:string)  [unwired: 3 in]
            }
            frame "M_EmA2dCalData.M_BipLowVoltPrimary.M_Offset" {
              n173 = Unbundle By Name(w464) -> ("M_EmA2dCalData.M_BipLowVoltPrimary.M_Offset"=w462:dbl)
              n174 = Number To Fractional String(number=w462) -> (F-format string=w461:string)  [unwired: 3 in]
            }
            frame "M_EmA2dCalData.M_BipLowVoltPrimary.M_Gain" {
              n175 = Unbundle By Name(w468) -> ("M_EmA2dCalData.M_BipLowVoltPrimary.M_Gain"=w466:dbl)
              n176 = Number To Fractional String(number=w466) -> (F-format string=w465:string)  [unwired: 3 in]
            }
            frame "M_EmA2dCalData.M_BipLowVoltSecondary.M_Offset" {
              n177 = Unbundle By Name(w472) -> ("M_EmA2dCalData.M_BipLowVoltSecondary.M_Offset"=w470:dbl)
              n178 = Number To Fractional String(number=w470) -> (F-format string=w469:string)  [unwired: 3 in]
            }
            frame "M_EmA2dCalData.M_BipLowVoltSecondary.M_Gain" {
              n179 = Unbundle By Name(w476) -> ("M_EmA2dCalData.M_BipLowVoltSecondary.M_Gain"=w474:dbl)
              n180 = Number To Fractional String(number=w474) -> (F-format string=w473:string)  [unwired: 3 in]
            }
            frame "M_EmA2dCalData.M_BipHighVoltPrimary.M_Offset" {
              n181 = Unbundle By Name(w480) -> ("M_EmA2dCalData.M_BipHighVoltPrimary.M_Offset"=w478:dbl)
              n182 = Number To Fractional String(number=w478) -> (F-format string=w477:string)  [unwired: 3 in]
            }
            frame "M_EmA2dCalData.M_BipHighVoltPrimary.M_Gain" {
              n183 = Unbundle By Name(w484) -> ("M_EmA2dCalData.M_BipHighVoltPrimary.M_Gain"=w482:dbl)
              n184 = Number To Fractional String(number=w482) -> (F-format string=w481:string)  [unwired: 3 in]
            }
            frame "M_EmA2dCalData.M_BipHighVoltSecondary.M_Offset" {
              n185 = Unbundle By Name(w488) -> ("M_EmA2dCalData.M_BipHighVoltSecondary.M_Offset"=w486:dbl)
              n186 = Number To Fractional String(number=w486) -> (F-format string=w485:string)  [unwired: 3 in]
            }
            frame "M_EmA2dCalData.M_BipHighVoltSecondary.M_Gain" {
              n187 = Unbundle By Name(w492) -> ("M_EmA2dCalData.M_BipHighVoltSecondary.M_Gain"=w490:dbl)
              n188 = Number To Fractional String(number=w490) -> (F-format string=w489:string)  [unwired: 3 in]
            }
            frame "M_EmA2dCalData.M_BipLowCurrentPrimary.M_Offset" {
              n189 = Unbundle By Name(w496) -> ("M_EmA2dCalData.M_BipLowCurrentPrimary.M_Offset"=w494:dbl)
              n190 = Number To Fractional String(number=w494) -> (F-format string=w493:string)  [unwired: 3 in]
            }
            frame "M_EmA2dCalData.M_BipLowCurrentPrimary.M_Gain" {
              n191 = Unbundle By Name(w500) -> ("M_EmA2dCalData.M_BipLowCurrentPrimary.M_Gain"=w498:dbl)
              n192 = Number To Fractional String(number=w498) -> (F-format string=w497:string)  [unwired: 3 in]
            }
            frame "M_EmA2dCalData.M_BipLowCurrentSecondary.M_Offset" {
              n193 = Unbundle By Name(w504) -> ("M_EmA2dCalData.M_BipLowCurrentSecondary.M_Offset"=w502:dbl)
              n194 = Number To Fractional String(number=w502) -> (F-format string=w501:string)  [unwired: 3 in]
            }
            frame "M_EmA2dCalData.M_BipLowCurrentSecondary.M_Gain" {
              n195 = Unbundle By Name(w508) -> ("M_EmA2dCalData.M_BipLowCurrentSecondary.M_Gain"=w506:dbl)
              n196 = Number To Fractional String(number=w506) -> (F-format string=w505:string)  [unwired: 3 in]
            }
            frame "M_EmA2dCalData.M_BipHighCurrentPrimary.M_Offset" {
              n197 = Unbundle By Name(w512) -> ("M_EmA2dCalData.M_BipHighCurrentPrimary.M_Offset"=w510:dbl)
              n198 = Number To Fractional String(number=w510) -> (F-format string=w509:string)  [unwired: 3 in]
            }
            frame "M_EmA2dCalData.M_BipHighCurrentPrimary.M_Gain" {
              n199 = Unbundle By Name(w516) -> ("M_EmA2dCalData.M_BipHighCurrentPrimary.M_Gain"=w514:dbl)
              n200 = Number To Fractional String(number=w514) -> (F-format string=w513:string)  [unwired: 3 in]
            }
            frame "M_EmA2dCalData.M_BipHighCurrentSecondary.M_Offset" {
              n201 = Unbundle By Name(w520) -> ("M_EmA2dCalData.M_BipHighCurrentSecondary.M_Offset"=w518:dbl)
              n202 = Number To Fractional String(number=w518) -> (F-format string=w517:string)  [unwired: 3 in]
            }
            frame "M_EmA2dCalData.M_BipHighCurrentSecondary.M_Gain" {
              n203 = Unbundle By Name(w524) -> ("M_EmA2dCalData.M_BipHighCurrentSecondary.M_Gain"=w522:dbl)
              n204 = Number To Fractional String(number=w522) -> (F-format string=w521:string)  [unwired: 3 in]
            }
            frame "ErrorStatus" {
              n205 = Select(t="Error", s=w525, f="Success") -> (s? t:f=w526:string)
            }
          }
        }
        frame "ExternalCommCommand" {
          n206 = Unflatten From JSON(JSON string=w533, type and defaults=T23 {"Partition"="", "Message"="", "M_ControllerBoardId"="", "M_ChassisSerialNumber"="", "M_Alias"="", "M_PrimaryIpAddress"="", "M_PairingStatus"=3, "M_PairedEntityIpAddress"="", "M_PairedEntityAlias"="", "M_PairedEntityId"="", "M_Options"="", "M_DftMode"=0, "M_IsViperEnabled"=TRUE}, default null elements? (F)=TRUE, error in (no error)=w538) -> (value=w534:T23, error out=w536:errorcluster)  [unwired: 3 in]
          n207 = case shown="\"ErrorStatus\"" w535 {
            tunnel: w536 -> [w539 w541 w544 w547 w550 w553 w556 w565 w567 w570 w573 w576 w583 w591 w593]
            tunnel: w534 -> [_ w543 w546 w549 w552 w555 w558 w566 w569 w572 w575 w578 w586 w592 _]
            tunnel: w533 -> [w540 _ _ _ _ _ _ _ _ _ _ _ _ _ _]
            tunnel: [w540 w542 w545 w548 w551 w554 w557 w559 w568 w571 w574 w577 w581 w587 w594] -> w532
            tunnel: [w539 w541 w544 w547 w550 w553 w556 w564 w567 w570 w573 w576 w582 w591 w593] -> w531
            tunnel: w530 -> [_ _ _ _ _ _ _ w561 _ _ _ _ w579 _ _]
            frame "All", Default {
            }
            frame "Partition" {
              n208 = Unbundle By Name(w543) -> ("Partition"=w542:string)
            }
            frame "Message" {
              n209 = Unbundle By Name(w546) -> ("Message"=w545:string)
            }
            frame "M_ControllerBoardId" {
              n210 = Unbundle By Name(w549) -> ("M_ControllerBoardId"=w548:string)
            }
            frame "M_ChassisSerialNumber" {
              n211 = Unbundle By Name(w552) -> ("M_ChassisSerialNumber"=w551:string)
            }
            frame "M_Alias" {
              n212 = Unbundle By Name(w555) -> ("M_Alias"=w554:string)
            }
            frame "M_PrimaryIpAddress" {
              n213 = Unbundle By Name(w558) -> ("M_PrimaryIpAddress"=w557:string)
            }
            frame "M_PairingStatus" {
              n214 = Unbundle By Name(w566) -> ("M_PairingStatus"=w562:T10)
              n215 = Number To Decimal String(number=w562) -> (decimal integer string=w560:string)  [unwired: 1 in]
              n216 = property on="ExternalCommPairingStatus" class="Ring (strict)"(error in=w565, "Value"=w562) -> (error out=w564:errorcluster, "RingText.Text"=w563:string)  [unwired: 1 in, 1 out]
              n217 = Select(t=w563, s=w561, f=w560) -> (s? t:f=w559:string)
            }
            frame "M_PairedEntityIpAddress" {
              n218 = Unbundle By Name(w569) -> ("M_PairedEntityIpAddress"=w568:string)
            }
            frame "M_PairedEntityAlias" {
              n219 = Unbundle By Name(w572) -> ("M_PairedEntityAlias"=w571:string)
            }
            frame "M_PairedEntityId" {
              n220 = Unbundle By Name(w575) -> ("M_PairedEntityId"=w574:string)
            }
            frame "M_Options" {
              n221 = Unbundle By Name(w578) -> ("M_Options"=w577:string)
            }
            frame "M_DftMode" {
              n222 = Unbundle By Name(w586) -> ("M_DftMode"=w580:T9)
              n223 = Number To Decimal String(number=w580) -> (decimal integer string=w584:string)  [unwired: 1 in]
              n224 = property on="DftMode" class="Ring (strict)"(error in=w583, "Value"=w580) -> (error out=w582:errorcluster, "RingText.Text"=w585:string)  [unwired: 1 in, 1 out]
              n225 = Select(t=w585, s=w579, f=w584) -> (s? t:f=w581:string)
            }
            frame "M_IsViperEnabled" {
              n226 = Unbundle By Name(w592) -> ("M_IsViperEnabled"=w590:bool)
              n227 = Select(t="TRUE", s=w590, f="FALSE") -> (s? t:f=w587:string)
            }
            frame "ErrorStatus" {
              n228 = Select(t="Error", s=w593, f="Success") -> (s? t:f=w594:string)
            }
          }
        }
        frame "FeatureSettingsCommand" {
          n229 = Unflatten From JSON(JSON string=w601, type and defaults=T24 {"Partition"="", "Message"="", "M_DisplayOrder"=0, "M_FeatureSetting"=0, "M_FeatureSettingName"="", "M_FeatureStatus"=0, "M_FeatureStatusText"="", "M_IntValue"=0, "M_IsEnablable"=TRUE, "M_IsEnabled"=TRUE, "M_IsEntitled"=TRUE, "M_IsEntitlable"=TRUE, "M_LastEnabledUpdate"=0, "M_LastEntitledUpdate"=0, "M_LicenseKey"="", "M_LicenseTerms"="", "M_Options"="", "M_StringValue"=""}, default null elements? (F)=TRUE, error in (no error)=w606) -> (value=w602:T24, error out=w604:errorcluster)  [unwired: 3 in]
          n230 = case shown="\"ErrorStatus\"" w603 {
            tunnel: w604 -> [w607 w609 w612 w617 w621 w623 w628 w630 w635 w641 w647 w653 w659 w663 w667 w669 w672 w675 w678 w681]
            tunnel: w602 -> [_ w611 w614 w618 w622 w625 w629 w632 w636 w642 w648 w654 w660 w664 w668 w671 w674 w677 w680 _]
            tunnel: w601 -> [w608 _ _ _ _ _ _ _ _ _ _ _ _ _ _ _ _ _ _ _]
            tunnel: [w608 w610 w613 w615 w619 w624 w626 w631 w633 w637 w643 w649 w655 w661 w665 w670 w673 w676 w679 w682] -> w600
            tunnel: [w607 w609 w612 w617 w621 w623 w628 w630 w635 w641 w647 w653 w659 w663 w667 w669 w672 w675 w678 w681] -> w599
            tunnel: w598 -> [_ _ _ _ _ _ _ _ _ _ _ _ _ _ _ _ _ _ _ _]
            frame "All", Default {
            }
            frame "Partition" {
              n231 = Unbundle By Name(w611) -> ("Partition"=w610:string)
            }
            frame "Message" {
              n232 = Unbundle By Name(w614) -> ("Message"=w613:string)
            }
            frame "M_DisplayOrder" {
              n233 = Unbundle By Name(w618) -> ("M_DisplayOrder"=w616:i32)
              n234 = Number To Decimal String(number=w616) -> (decimal integer string=w615:string)  [unwired: 1 in]
            }
            frame "M_FeatureSetting" {
              n235 = Unbundle By Name(w622) -> ("M_FeatureSetting"=w620:i32)
              n236 = Number To Decimal String(number=w620) -> (decimal integer string=w619:string)  [unwired: 1 in]
            }
            frame "M_FeatureSettingName" {
              n237 = Unbundle By Name(w625) -> ("M_FeatureSettingName"=w624:string)
            }
            frame "M_FeatureStatus" {
              n238 = Unbundle By Name(w629) -> ("M_FeatureStatus"=w627:i32)
              n239 = Number To Decimal String(number=w627) -> (decimal integer string=w626:string)  [unwired: 1 in]
            }
            frame "M_FeatureStatusText" {
              n240 = Unbundle By Name(w632) -> ("M_FeatureStatusText"=w631:string)
            }
            frame "M_IntValue" {
              n241 = Unbundle By Name(w636) -> ("M_IntValue"=w634:i32)
              n242 = Number To Decimal String(number=w634) -> (decimal integer string=w633:string)  [unwired: 1 in]
            }
            frame "M_IsEnablable" {
              n243 = Unbundle By Name(w642) -> ("M_IsEnablable"=w640:bool)
              n244 = Select(t="TRUE", s=w640, f="FALSE") -> (s? t:f=w637:string)
            }
            frame "M_IsEnabled" {
              n245 = Unbundle By Name(w648) -> ("M_IsEnabled"=w646:bool)
              n246 = Select(t="TRUE", s=w646, f="FALSE") -> (s? t:f=w643:string)
            }
            frame "M_IsEntitled" {
              n247 = Unbundle By Name(w654) -> ("M_IsEntitled"=w652:bool)
              n248 = Select(t="TRUE", s=w652, f="FALSE") -> (s? t:f=w649:string)
            }
            frame "M_IsEntitlable" {
              n249 = Unbundle By Name(w660) -> ("M_IsEntitlable"=w658:bool)
              n250 = Select(t="TRUE", s=w658, f="FALSE") -> (s? t:f=w655:string)
            }
            frame "M_LastEnabledUpdate" {
              n251 = Unbundle By Name(w664) -> ("M_LastEnabledUpdate"=w662:i32)
              n252 = Number To Decimal String(number=w662) -> (decimal integer string=w661:string)  [unwired: 1 in]
            }
            frame "M_LastEntitledUpdate" {
              n253 = Unbundle By Name(w668) -> ("M_LastEntitledUpdate"=w666:i32)
              n254 = Number To Decimal String(number=w666) -> (decimal integer string=w665:string)  [unwired: 1 in]
            }
            frame "M_LicenseKey" {
              n255 = Unbundle By Name(w671) -> ("M_LicenseKey"=w670:string)
            }
            frame "M_LicenseTerms" {
              n256 = Unbundle By Name(w674) -> ("M_LicenseTerms"=w673:string)
            }
            frame "M_Options" {
              n257 = Unbundle By Name(w677) -> ("M_Options"=w676:string)
            }
            frame "M_StringValue" {
              n258 = Unbundle By Name(w680) -> ("M_StringValue"=w679:string)
            }
            frame "ErrorStatus" {
              n259 = Select(t="Error", s=w681, f="Success") -> (s? t:f=w682:string)
            }
          }
        }
        frame "SystemConfigurationCommand" {
          n260 = case shown="\"ErrorStatus\"" w690 {
            tunnel: w685 -> [w691 w693]
            tunnel: w689 -> [w692 _]
            tunnel: [w692 w694] -> w688
            tunnel: [w691 w693] -> w687
            tunnel: w686 -> [_ _]
            frame "All", Default {
            }
            frame "ErrorStatus" {
              n261 = Select(t="Error", s=w693, f="Success") -> (s? t:f=w694:string)
            }
          }
        }
        frame "SupervisorCommand" {
          n262 = case shown="\"ErrorStatus\"" w702 {
            tunnel: w697 -> [w703 w705]
            tunnel: w701 -> [w704 _]
            tunnel: [w704 w706] -> w700
            tunnel: [w703 w705] -> w699
            tunnel: w698 -> [_ _]
            frame "All", Default {
            }
            frame "ErrorStatus" {
              n263 = Select(t="Error", s=w705, f="Success") -> (s? t:f=w706:string)
            }
          }
        }
        frame "SystemSettingsCommand" {
          n264 = Unflatten From JSON(JSON string=w713, type and defaults=T25 {"Partition"="", "Message"="", "M_SystemSetting"=0, "M_IntValue"=0, "M_StringValue"=""}, default null elements? (F)=TRUE, error in (no error)=w718) -> (value=w714:T25, error out=w716:errorcluster)  [unwired: 3 in]
          n265 = case shown="\"All\", Default" w715 {
            tunnel: w716 -> [w719 w721 w724 w733 w737 w739 w742]
            tunnel: w714 -> [_ w723 w726 w734 w738 w741 _]
            tunnel: w713 -> [w720 _ _ _ _ _ _]
            tunnel: [w720 w722 w725 w727 w735 w740 w743] -> w712
            tunnel: [w719 w721 w724 w732 w737 w739 w742] -> w711
            tunnel: w710 -> [_ _ _ w729 _ _ _]
            frame "All", Default {
            }
            frame "Partition" {
              n266 = Unbundle By Name(w723) -> ("Partition"=w722:string)
            }
            frame "Message" {
              n267 = Unbundle By Name(w726) -> ("Message"=w725:string)
            }
            frame "M_SystemSetting" {
              n268 = Unbundle By Name(w734) -> ("M_SystemSetting"=w730:T8)
              n269 = Number To Decimal String(number=w730) -> (decimal integer string=w728:string)  [unwired: 1 in]
              n270 = property on="SystemSettings" class="Ring (strict)"(error in=w733, "Value"=w730) -> (error out=w732:errorcluster, "RingText.Text"=w731:string)  [unwired: 1 in, 1 out]
              n271 = Select(t=w731, s=w729, f=w728) -> (s? t:f=w727:string)
            }
            frame "M_IntValue" {
              n272 = Unbundle By Name(w738) -> ("M_IntValue"=w736:i32)
              n273 = Number To Decimal String(number=w736) -> (decimal integer string=w735:string)  [unwired: 1 in]
            }
            frame "M_StringValue" {
              n274 = Unbundle By Name(w741) -> ("M_StringValue"=w740:string)
            }
            frame "ErrorStatus" {
              n275 = Select(t="Error", s=w742, f="Success") -> (s? t:f=w743:string)
            }
          }
        }
        frame "TimeCommand" {
          n276 = Unflatten From JSON(JSON string=w750, type and defaults=T26 {"Partition"="", "Message"="", "M_UtcTime"="", "M_LocalTime"="", "M_TimeZone"=""}, default null elements? (F)=TRUE, error in (no error)=w755) -> (value=w751:T26, error out=w753:errorcluster)  [unwired: 3 in]
          n277 = case shown="\"ErrorStatus\"" w752 {
            tunnel: w753 -> [w756 w758 w761 w764 w767 w770 w773]
            tunnel: w751 -> [_ w760 w763 w766 w769 w772 _]
            tunnel: w750 -> [w757 _ _ _ _ _ _]
            tunnel: [w757 w759 w762 w765 w768 w771 w774] -> w749
            tunnel: [w756 w758 w761 w764 w767 w770 w773] -> w748
            tunnel: w747 -> [_ _ _ _ _ _ _]
            frame "All", Default {
            }
            frame "Partition" {
              n278 = Unbundle By Name(w760) -> ("Partition"=w759:string)
            }
            frame "Message" {
              n279 = Unbundle By Name(w763) -> ("Message"=w762:string)
            }
            frame "M_UtcTime" {
              n280 = Unbundle By Name(w766) -> ("M_UtcTime"=w765:string)
            }
            frame "M_LocalTime" {
              n281 = Unbundle By Name(w769) -> ("M_LocalTime"=w768:string)
            }
            frame "M_TimeZone" {
              n282 = Unbundle By Name(w772) -> ("M_TimeZone"=w771:string)
            }
            frame "ErrorStatus" {
              n283 = Select(t="Error", s=w773, f="Success") -> (s? t:f=w774:string)
            }
          }
        }
        frame "UserSettingsCommand" {
          n284 = Unflatten From JSON(JSON string=w781, type and defaults=T27 {"Partition"="", "Message"="", "M_UserSetting"=0, "M_IntValue"=0, "M_StringValue"=""}, default null elements? (F)=TRUE, error in (no error)=w786) -> (value=w782:T27, error out=w784:errorcluster)  [unwired: 3 in]
          n285 = case shown="\"ErrorStatus\"" w783 {
            tunnel: w784 -> [w787 w789 w792 w801 w805 w807 w810]
            tunnel: w782 -> [_ w791 w794 w802 w806 w809 _]
            tunnel: w781 -> [w788 _ _ _ _ _ _]
            tunnel: [w788 w790 w793 w795 w803 w808 w811] -> w780
            tunnel: [w787 w789 w792 w800 w805 w807 w810] -> w779
            tunnel: w778 -> [_ _ _ w797 _ _ _]
            frame "All", Default {
            }
            frame "Partition" {
              n286 = Unbundle By Name(w791) -> ("Partition"=w790:string)
            }
            frame "Message" {
              n287 = Unbundle By Name(w794) -> ("Message"=w793:string)
            }
            frame "M_UserSetting" {
              n288 = Unbundle By Name(w802) -> ("M_UserSetting"=w798:T7)
              n289 = Number To Decimal String(number=w798) -> (decimal integer string=w796:string)  [unwired: 1 in]
              n290 = property on="UserSettings" class="Ring (strict)"(error in=w801, "Value"=w798) -> (error out=w800:errorcluster, "RingText.Text"=w799:string)  [unwired: 1 in, 1 out]
              n291 = Select(t=w799, s=w797, f=w796) -> (s? t:f=w795:string)
            }
            frame "M_IntValue" {
              n292 = Unbundle By Name(w806) -> ("M_IntValue"=w804:i32)
              n293 = Number To Decimal String(number=w804) -> (decimal integer string=w803:string)  [unwired: 1 in]
            }
            frame "M_StringValue" {
              n294 = Unbundle By Name(w809) -> ("M_StringValue"=w808:string)
            }
            frame "ErrorStatus" {
              n295 = Select(t="Error", s=w810, f="Success") -> (s? t:f=w811:string)
            }
          }
        }
        frame "VolumeBarsCommand" {
          n296 = Unflatten From JSON(JSON string=w818, type and defaults=T28 {"Partition"="", "Message"="", "M_VolumeBars"=0, "M_RangeState"=0, "M_VolumeCloseOverlay"=TRUE}, default null elements? (F)=TRUE, error in (no error)=w823) -> (value=w819:T28, error out=w821:errorcluster)  [unwired: 3 in]
          n297 = case shown="\"M_RangeState\"" w820 {
            tunnel: w821 -> [w824 w826 w829 w838 w842 w848 w850]
            tunnel: w819 -> [_ w828 w831 w839 w843 w849 _]
            tunnel: w818 -> [w825 _ _ _ _ _ _]
            tunnel: [w825 w827 w830 w832 w840 w844 w851] -> w817
            tunnel: [w824 w826 w829 w837 w842 w848 w850] -> w816
            tunnel: w815 -> [_ _ _ w834 _ _ _]
            frame "All", Default {
            }
            frame "Partition" {
              n298 = Unbundle By Name(w828) -> ("Partition"=w827:string)
            }
            frame "Message" {
              n299 = Unbundle By Name(w831) -> ("Message"=w830:string)
            }
            frame "M_RangeState" {
              n300 = Unbundle By Name(w839) -> ("M_RangeState"=w835:T14)
              n301 = Number To Decimal String(number=w835) -> (decimal integer string=w833:string)  [unwired: 1 in]
              n302 = property on="ParameterRangeState" class="Ring (strict)"(error in=w838, "Value"=w835) -> (error out=w837:errorcluster, "RingText.Text"=w836:string)  [unwired: 1 in, 1 out]
              n303 = Select(t=w836, s=w834, f=w833) -> (s? t:f=w832:string)
            }
            frame "M_VolumeBars" {
              n304 = Unbundle By Name(w843) -> ("M_VolumeBars"=w841:i32)
              n305 = Number To Decimal String(number=w841) -> (decimal integer string=w840:string)  [unwired: 1 in]
            }
            frame "M_VolumeCloseOverlay" {
              n306 = Unbundle By Name(w849) -> ("M_VolumeCloseOverlay"=w847:bool)
              n307 = Select(t="TRUE", s=w847, f="FALSE") -> (s? t:f=w844:string)
            }
            frame "ErrorStatus" {
              n308 = Select(t="Error", s=w850, f="Success") -> (s? t:f=w851:string)
            }
          }
        }
        frame "ViperCmd" {
          n309 = global read "S2C_FORNAX_Proc_Globals.vi" "Version"() -> (w854:i32)
          n310 = case shown="1, Default" w854 {
            tunnel: w860 -> [w870 w899]
            tunnel: w859 -> [w867 w896]
            tunnel: w858 -> [w865 w894]
            tunnel: [w864 w893] -> w857
            tunnel: [w863 w892] -> w856
            tunnel: w855 -> [w862 w891]
            frame 1, Default {
              n311 = Unflatten From JSON(JSON string=w865, type and defaults=T29 {"Partition"="", "Message"="", "M_ViperMessage"="", "M_SrcId"=0}, default null elements? (F)=TRUE, error in (no error)=w870) -> (value=w866:T29, error out=w868:errorcluster)  [unwired: 3 in]
              n312 = case shown="\"Message\"" w867 {
                tunnel: w868 -> [w871 w873 w876 w879 w884 w886]
                tunnel: w866 -> [_ w875 w878 w881 w885 _]
                tunnel: w865 -> [w872 _ _ _ _ _]
                tunnel: [w872 w874 w877 w880 w882 w887] -> w864
                tunnel: [w871 w873 w876 w879 w884 w886] -> w863
                tunnel: w862 -> [_ _ _ _ _ _]
                frame "All", Default {
                }
                frame "Partition" {
                  n313 = Unbundle By Name(w875) -> ("Partition"=w874:string)
                }
                frame "Message" {
                  n314 = Unbundle By Name(w878) -> ("Message"=w877:string)
                }
                frame "M_message" {
                  n315 = Unbundle By Name(w881) -> ("M_ViperMessage"=w880:string)
                }
                frame "M_srcId" {
                  n316 = Unbundle By Name(w885) -> ("M_SrcId"=w883:i32)
                  n317 = Number To Decimal String(number=w883) -> (decimal integer string=w882:string)  [unwired: 1 in]
                }
                frame "ErrorStatus" {
                  n318 = Select(t="Error", s=w886, f="Success") -> (s? t:f=w887:string)
                }
              }
            }
            frame 3 {
              n319 = Unflatten From JSON(JSON string=w894, type and defaults=T30 {"Partition"="", "Message"="", "M_message"="", "M_srcId"=0}, default null elements? (F)=TRUE, error in (no error)=w899) -> (value=w895:T30, error out=w897:errorcluster)  [unwired: 3 in]
              n320 = case shown="\"ErrorStatus\"" w896 {
                tunnel: w897 -> [w900 w902 w905 w908 w913 w915]
                tunnel: w895 -> [_ w904 w907 w910 w914 _]
                tunnel: w894 -> [w901 _ _ _ _ _]
                tunnel: [w901 w903 w906 w909 w911 w916] -> w893
                tunnel: [w900 w902 w905 w908 w913 w915] -> w892
                tunnel: w891 -> [_ _ _ _ _ _]
                frame "All", Default {
                }
                frame "Partition" {
                  n321 = Unbundle By Name(w904) -> ("Partition"=w903:string)
                }
                frame "Message" {
                  n322 = Unbundle By Name(w907) -> ("Message"=w906:string)
                }
                frame "M_message" {
                  n323 = Unbundle By Name(w910) -> ("M_message"=w909:string)
                }
                frame "M_srcId" {
                  n324 = Unbundle By Name(w914) -> ("M_srcId"=w912:i32)
                  n325 = Number To Decimal String(number=w912) -> (decimal integer string=w911:string)  [unwired: 1 in]
                }
                frame "ErrorStatus" {
                  n326 = Select(t="Error", s=w915, f="Success") -> (s? t:f=w916:string)
                }
              }
            }
          }
        }
      }
      n327 = call <vilib>:"Trim Whitespace.vi"("string"=w6) -> ("trimmed string"=→"Data":string)  [unwired: 1 in]
    }
    frame Error {
    }
  }
  "Error Out" <- w1
